vi "File Configuration.vi"(8 "error in":errorcluster, 10 "Calibration Configuration":T1, 11 "Logging Configuration in":T2) -> (0 "error out":errorcluster, 3 "Logging Configuration out":T2)   [LabVIEW 2024]
uses:
  Logging Configuration.ctl
  Configuration/Calibration Configuration.ctl
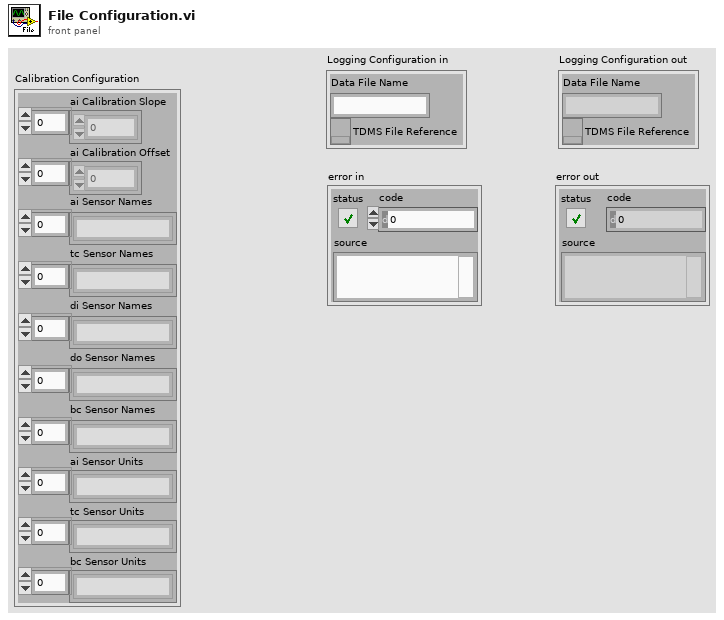
[diagram p1: front panel]
types:
  T1 = typedef "Calibration Configuration.ctl" = cluster{"ai Calibration Slope":dbl[], "ai Calibration Offset":dbl[], "ai Sensor Names ":string[], "tc Sensor Names":string[], "di Sensor Names":string[], "do Sensor Names":string[], "bc Sensor Names":string[], "ai Sensor Units":string[], "tc Sensor Units":string[], "bc Sensor Units":string[]}
  T2 = typedef "Logging Configuration.ctl" = cluster{"Data File Name":string, "TDMS File Reference":refnum<k34>}
  T3 = enum16{"open", "open or create", "create or replace", "create", "open (read-only)"}
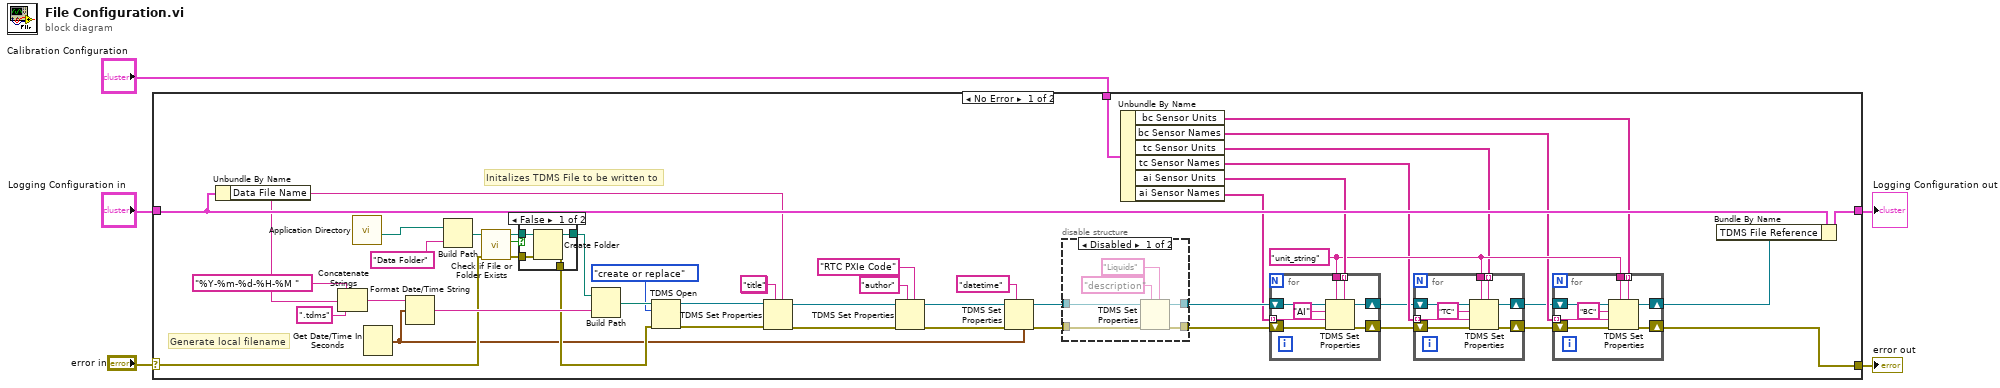
[diagram p0: block diagram]
diagram:
  n1 = case shown="No Error" "error in" {
    selector: "error in" -> [w37 w92]
    tunnel: "Logging Configuration in" -> [w46 w91]
    tunnel: [w10 w92] -> w3
    tunnel: [w45 w91] -> w2
    tunnel: "Calibration Configuration" -> [w20 _]
    frame No Error {
      w17 = "unit_string"
      (unwired) "title"
      # "Initalizes TDMS File to be written to"
      # "Generate local filename"
      n2 = Unbundle By Name(w46) -> ("Data File Name"=w23:string)
      n3 = Concatenate Strings("%Y-%m-%d-%H-%M ", w23, ".tdms") -> (w49:string)
      n4 = call <vilib>:"Application Directory.vi"() -> ("Application Directory"=w43:path)
      n5 = Get Date/Time In Seconds() -> (seconds since 1Jan1904=w22:timestamp)
      n6 = Format Date/Time String(time format string (%c)=w49, seconds (now)=w22) -> (date/time string=w52:string)  [unwired: 1 in]
      n7 = Build Path(base path=w43, name or relative path="Data Folder") -> (appended path=w42:path)
      n8 = call <vilib>:"Check if File or Folder Exists.vi"("error in (no error)"=w37, "path"=w42) -> ("error out"=w38:errorcluster, "file or folder exists?"=w39:bool, "dup path"=w41:path)  [unwired: 7 in]
      n9 = case shown="False" w39 {
        tunnel: w41 -> [w88 w90]
        tunnel: [w87 w90] -> w40
        tunnel: w38 -> [w86 w89]
        tunnel: [w85 w89] -> w36
        frame False {
          n10 = Create Folder(path (use dialog)=w88, error in=w86) -> (created path=w87:path, error out=w85:errorcluster)  [unwired: 1 in, 1 out]
        }
        frame True {
        }
      }
      n11 = Build Path(base path=w40, name or relative path=w52) -> (appended path=w47:path)
      n12 = TDMS Open(8:w36, 10:T3."create or replace" ("operation (0:open)"), 11:w47) -> (0:w24:errorcluster, 3:w25:refnum<k34>)  [unwired: 4 in]
      n13 = TDMS Set Properties(5:w23, 7:"title", 8:w24, 11:w25) -> (0:w31:errorcluster, 3:w30:refnum<k34>)  [unwired: 2 in, 2 out]
      n14 = TDMS Set Properties(5:"RTC PXIe Code", 7:"author", 8:w31, 11:w30) -> (0:w33:errorcluster, 3:w32:refnum<k34>)  [unwired: 2 in, 2 out]
      n15 = TDMS Set Properties(5:w22, 7:"datetime", 8:w33, 11:w32) -> (0:w35:errorcluster, 3:w34:refnum<k34>)  [unwired: 2 in, 2 out]
      n16 = disable-structure shown="Disabled" {
        disable-tunnel: w35 -> [w82 w83]
        disable-tunnel: w34 -> [w81 w84]
        disable-tunnel: [w78 w84] -> w21
        disable-tunnel: [w77 w83] -> w18
        frame Disabled {
          n17 = TDMS Set Properties(5:"Liquids", 7:"description", 8:w82, 11:w81) -> (0:w77:errorcluster, 3:w78:refnum<k34>)  [unwired: 2 in, 2 out]
        }
        frame Enabled {
        }
      }
      n18 = Unbundle By Name(w20) -> ("bc Sensor Units"=w16:string[], "bc Sensor Names"=w12:string[], "tc Sensor Units"=w15:string[], "tc Sensor Names"=w14:string[], "ai Sensor Units"=w19:string[], "ai Sensor Names"=w13:string[])
      n19 = for {
        tunnel: w13 -> [w71] mode=indexing
        shift-right: [w75] -> w7
        shift-left: w21 -> [w76]
        shift-right: [w73] -> w9
        shift-left: w18 -> [w74]
        tunnel: w19 -> [w70] mode=indexing
        tunnel: w17 -> [w69]
        n20 = TDMS Set Properties(5:w70, 7:w69, 8:w74, 9:w71, 10:"AI", 11:w76) -> (0:w73:errorcluster, 3:w75:refnum<k34>)  [unwired: 2 out]
      }
      n21 = for {
        tunnel: w14 -> [w63] mode=indexing
        shift-right: [w67] -> w6
        shift-left: w7 -> [w68]
        shift-right: [w65] -> w8
        shift-left: w9 -> [w66]
        tunnel: w15 -> [w62] mode=indexing
        tunnel: w17 -> [w61]
        n22 = TDMS Set Properties(5:w62, 7:w61, 8:w66, 9:w63, 10:"TC", 11:w68) -> (0:w65:errorcluster, 3:w67:refnum<k34>)  [unwired: 2 out]
      }
      n23 = for {
        tunnel: w12 -> [w55] mode=indexing
        shift-right: [w59] -> w11
        shift-left: w6 -> [w60]
        shift-right: [w57] -> w10
        shift-left: w8 -> [w58]
        tunnel: w16 -> [w54] mode=indexing
        tunnel: w17 -> [w53]
        n24 = TDMS Set Properties(5:w54, 7:w53, 8:w58, 9:w55, 10:"BC", 11:w60) -> (0:w57:errorcluster, 3:w59:refnum<k34>)  [unwired: 2 out]
      }
      n25 = Bundle By Name(cluster=w46, "TDMS File Reference"=w11) -> (w45:T2)
    }
    frame Error {
    }
  }
  "error out" <- w3
  "Logging Configuration out" <- w2
